vi "gl_UsrProfiles globals.vi"() -> ()   [LabVIEW 2020]
uses:
  Typedefs/User login window refs.ctl
panel:
  out "Right clicked on the loaded profile?":bool=TRUE
  out "Profile changed":bool
  in  "Loaded profile name":string
  in  "User logged in":string
  out "Selected profile to save":path
  out "New profile filepath":path
  in  "Copied profile":path
  out "User login window refs":T1
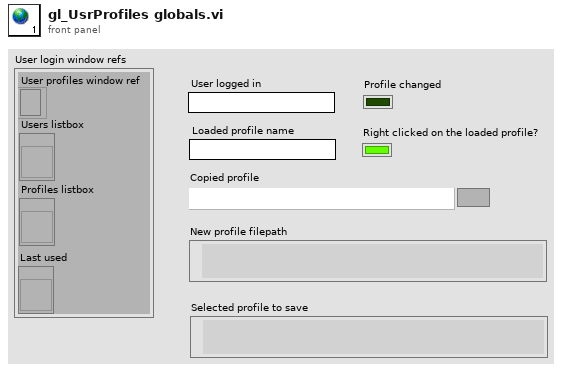
[diagram p1: front panel]
types:
  T1 = typedef "User login window refs.ctl" = cluster{"User profiles window ref":refnum<k9>, "Users listbox":refnum<vi>, "Profiles listbox":refnum<vi>, "Last used":refnum<vi>}
diagram:
